vi "T from SoS_AIR_v1_0_2025.vi"(0 "Max. n° iterations":i32=50, 1 "tolerance [mK]":dbl=0.05, 2 "cexp experimentally measured speed of sound [m/s]":dbl=343.9844 format="%.4f", 3 "initial T guess":dbl=300.0 format="%.3g", 4 "Pressure":dbl=1.0 format="%.3f", 6 "DT bisection start (degrees)":dbl=20.0 format="%.3g", 8 "Humidity":dbl=50.0 format="%.3g", 9 "Frequency":dbl=10.0) -> (7 "calculated acoustic Temperature Tcalc":dbl=293.14998626708984 format="%.4f")   [LabVIEW 2016]
panel:
  out "Temperature unit":i32(listbox)
  in  "Type of air":i32(listbox)=4
  in  "CO2 content (ppm)":dbl=500.0
  in  "frequency unit":i32(listbox)=1
  out "needed iterations":i32=19
  out "c(Tcalc) - cexp [m/s]":dbl=-3.994002895524318e-06 format="%.6f"
  out "calculated speed [m/s]":dbl=343.9843960059971 format="%.4f"
  in  "humidity unit":i32(listbox)=3
  in  "pressure unit":i32(listbox)=2
  in  "Temperature unit":i32(listbox)
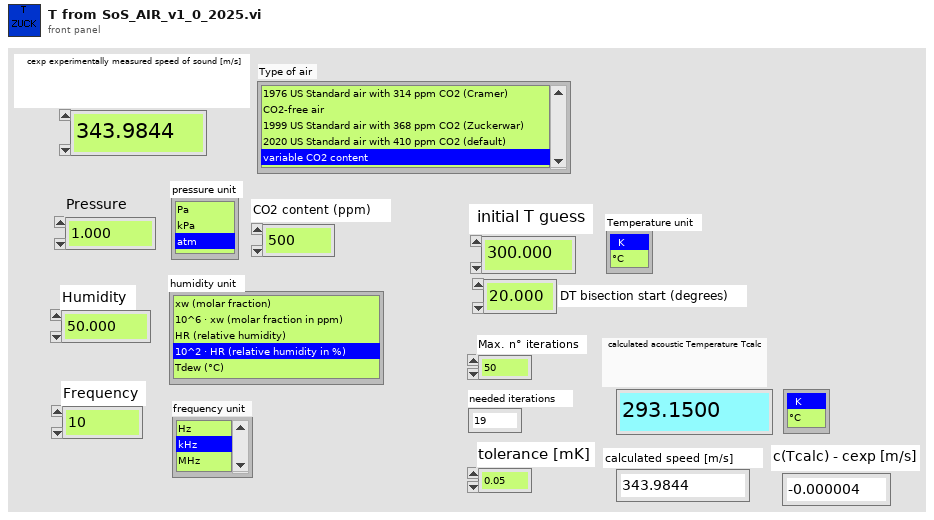
[diagram p1: front panel]
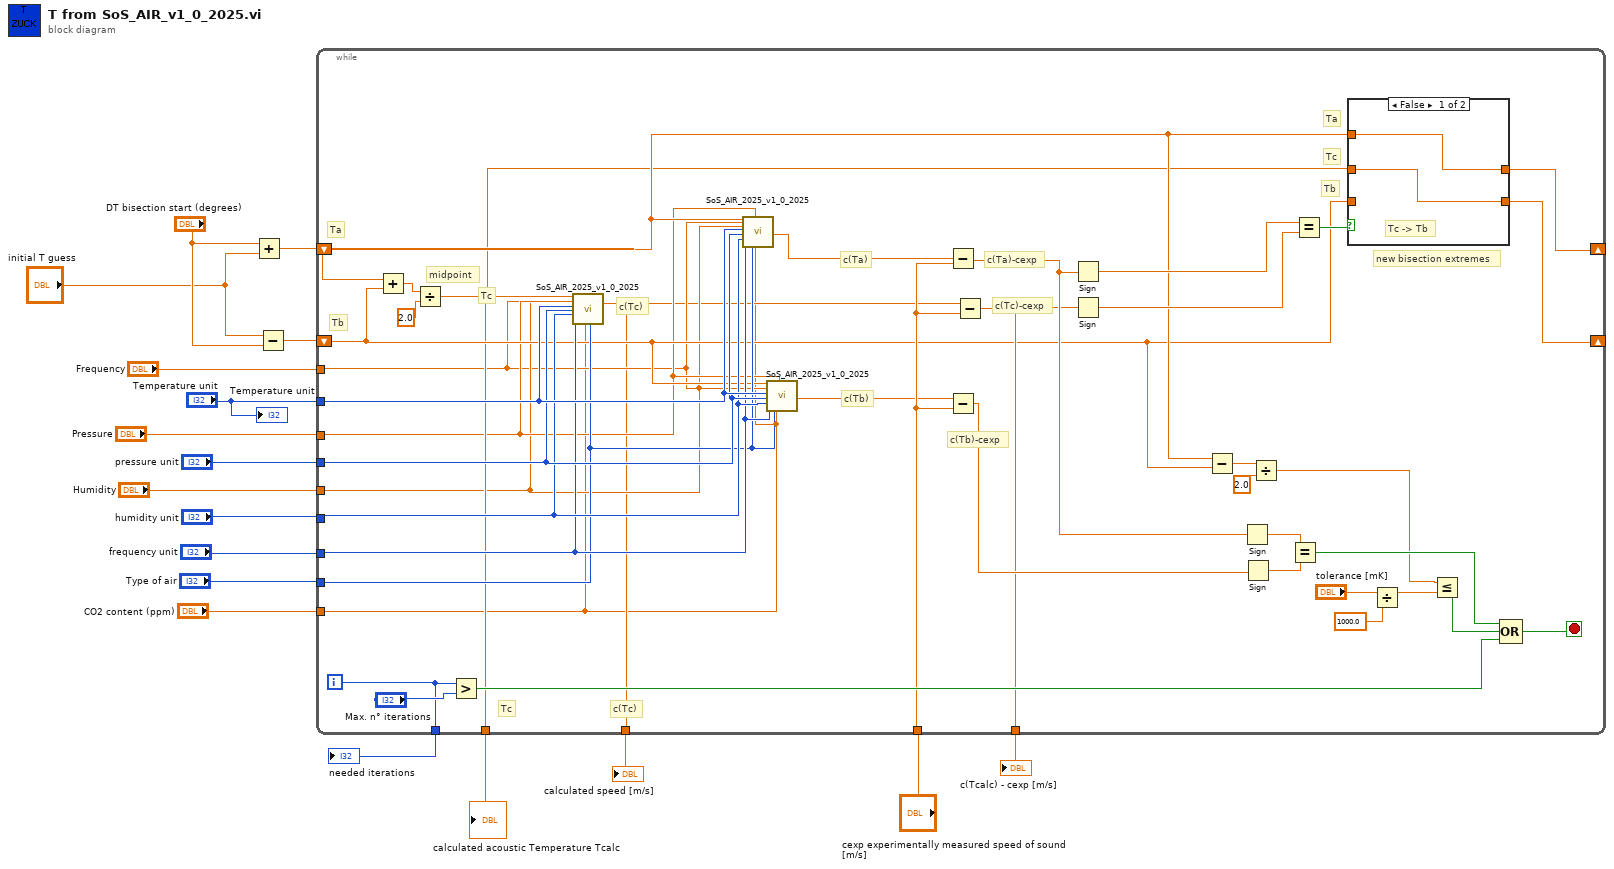
[diagram p0: block diagram]
diagram:
  n1 = Add(x="DT bisection start (degrees)", y="initial T guess") -> (x+y=w16:dbl)
  n2 = Subtract(x="initial T guess", y="DT bisection start (degrees)") -> (x-y=w15:dbl)
  n3 = while {
    tunnel: "cexp experimentally measured speed of sound [m/s]" -> [w44]
    shift-right: [w42] -> _
    shift-left: w16 -> [w28]
    shift-right: [w41] -> _
    shift-left: w15 -> [w27]
    tunnel: [w26] -> w13
    tunnel: [w20] -> w12
    tunnel: [w37] -> w11
    tunnel: [w34] -> w10
    tunnel: "Temperature unit" -> [w33]
    tunnel: "Pressure" -> [w25]
    tunnel: "Humidity" -> [w24]
    tunnel: "pressure unit" -> [w32]
    tunnel: "humidity unit" -> [w31]
    tunnel: "frequency unit" -> [w30]
    tunnel: "Type of air" -> [w29]
    tunnel: "Frequency" -> [w23]
    tunnel: "CO2 content (ppm)" -> [w19]
    i -> [w34]
    stop <- w50 stop-if-true
    # "Tc"
    # "c(Tc)"
    # "new bisection extremes"
    # "Tc"
    # "Tc"
    # "Tb"
    # "Ta"
    # "c(Tb)-cexp"
    # "c(Tc)-cexp"
    # "c(Ta)-cexp"
    # "c(Tc)"
    # "c(Tb)"
    # "c(Ta)"
    # "Tb"
    # "Ta"
    # "midpoint"
    n4 = Add(x=w28, y=w27) -> (x+y=w51:dbl)
    n5 = Divide(x=w51, y=2.0) -> (x/y=w26:dbl)
    n6 = Greater?(x=w34, y="Max. n° iterations") -> (0:w56:bool)
    n7 = call "SoS_AIR_2025_v1_0_2025.vi"("Temperature"=w26, "Frequency"=w23, "Temperature unit"=w33, "Pressure unit"=w32, "humidity unit"=w31, "frequency unit"=w30, "Humidity"=w24, "Type of air"=w29, "Pressure"=w25, "CO2 content / ppm"=w19) -> ("speed of sound humid air  [m/s]"=w20:dbl)  [unwired: 3 in, 6 out]
    n8 = call "SoS_AIR_2025_v1_0_2025.vi"("Temperature"=w28, "Frequency"=w23, "Temperature unit"=w33, "Pressure unit"=w32, "humidity unit"=w31, "frequency unit"=w30, "Humidity"=w24, "Type of air"=w29, "Pressure"=w25, "CO2 content / ppm"=w19) -> ("speed of sound humid air  [m/s]"=w21:dbl)  [unwired: 3 in, 6 out]
    n9 = call "SoS_AIR_2025_v1_0_2025.vi"("Temperature"=w27, "Frequency"=w23, "Temperature unit"=w33, "Pressure unit"=w32, "humidity unit"=w31, "frequency unit"=w30, "Humidity"=w24, "Type of air"=w29, "Pressure"=w25, "CO2 content / ppm"=w19) -> ("speed of sound humid air  [m/s]"=w22:dbl)  [unwired: 3 in, 6 out]
    n10 = Subtract(x=w21, y=w44) -> (x-y=w43:dbl)
    n11 = Subtract(x=w22, y=w44) -> (x-y=w52:dbl)
    n12 = Subtract(x=w20, y=w44) -> (x-y=w37:dbl)
    n13 = Sign(1:w43) -> (0:w40:dbl)
    n14 = Sign(1:w37) -> (0:w39:dbl)
    n15 = Subtract(x=w28, y=w27) -> (x-y=w47:dbl)
    n16 = Sign(1:w43) -> (0:w53:dbl)
    n17 = Sign(1:w52) -> (0:w54:dbl)
    n18 = Divide(x=w47, y=2.0) -> (x/y=w45:dbl)
    n19 = Equal?(x=w53, y=w54) -> (x = y?=w48:bool)
    n20 = Equal?(x=w40, y=w39) -> (x = y?=w38:bool)
    n21 = case shown="False" w38 {
      tunnel: w26 -> [w60 w62]
      tunnel: [w59 w62] -> w42
      tunnel: [w60 w61] -> w41
      tunnel: w28 -> [w59 _]
      tunnel: w27 -> [_ w61]
      frame False {
        # "Tc -> Tb"
      }
      frame True {
        # "Tc -> Ta"
      }
    }
    n22 = Divide(x="tolerance [mK]", y=1000.0) -> (x/y=w36:dbl)
    n23 = Less Or Equal?(x=w45, y=w36) -> (x <= y?=w55:bool)
    n24 = Compound Arithmetic op=OR(w48, w55, w56) -> (w50:bool)
  }
  "calculated acoustic Temperature Tcalc" <- w13
  "calculated speed [m/s]" <- w12
  "c(Tcalc) - cexp [m/s]" <- w11
  "needed iterations" <- w10
  "Temperature unit" <- "Temperature unit"
